vi "Read Main GUID.vi"(8 "Error In":errorcluster caption="error in", 11 "Custom Device .NET Ref In":refnum<k24>) -> (0 "Error out":errorcluster caption="error in", 2 "Main CD Properties":T1, 3 "Custom Device .NET Ref Out":refnum<k24>)   [LabVIEW 2019, in "VeriStand Custom Device XML Parser.lvlib"]
doc: "Reads and returns the main custom device properties"
uses:
  VeriStand Custom Device XML Parser.lvlib
  NationalInstruments.VeriStand.XMLReader
  XML Controls/Main Custom Device Properties.ctl
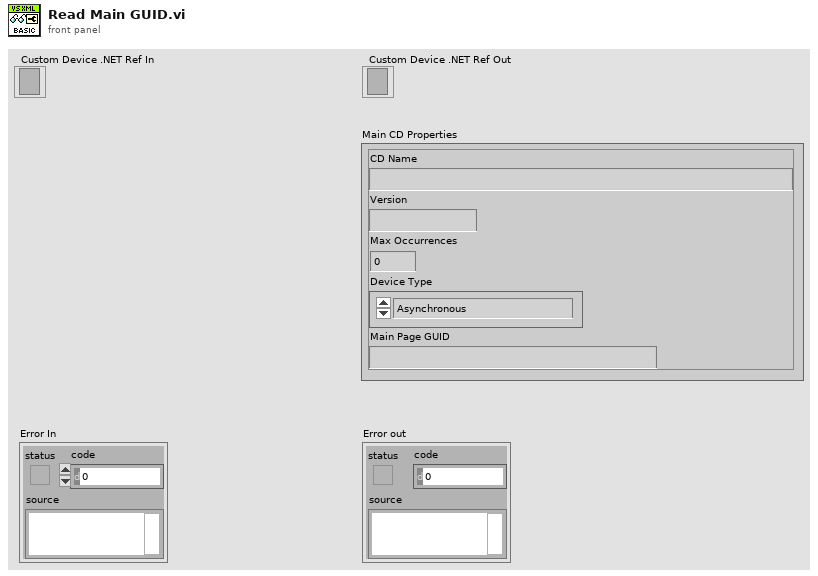
[diagram p1: front panel]
types:
  T1 = typedef "VeriStand Custom Device XML Parser.lvlib/Main Custom Device Properties.ctl" = cluster{"CD Name":string, "Version":string, "Max Occurrences":i32, "Device Type":enum16{"Asynchronous", "Inline HW Interface", "Inline Model Interface", "Inline Timing and Sync", "Asynchronous Timing and Sync"}, "Main Page GUID":string}
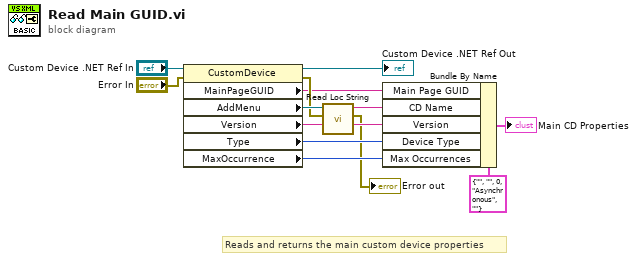
[diagram p0: block diagram]
diagram:
  # "Reads and returns the main custom device properties"
  n1 = property class="CustomDevice"(reference="Custom Device .NET Ref In", error in="Error In") -> (reference out=→"Custom Device .NET Ref Out":refnum<k24>, error out=w6:errorcluster, "MainPageGUID"=w2:string, "AddMenu"=w11:refnum<k24>, "Version"=w10:string, "Type"=w7:i32, "MaxOccurrence"=w9:i32)
  n2 = call "Read Loc String.vi"("Error In"=w6, "Loc String .NET Ref"=w11) -> ("Error Out"=→"Error out":errorcluster, "English"=w4:string)  [unwired: 7 in, 1 out]
  n3 = Bundle By Name(cluster=T1 {"CD Name"="", "Version"="", "Max Occurrences"=0, "Device Type"=enum."Asynchronous", "Main Page GUID"=""} ("Main CD Properties"), "Main Page GUID"=w2, "CD Name"=w4, "Version"=w10, "Device Type"=w7, "Max Occurrences"=w9) -> (→"Main CD Properties":T1)
